vi "Load Plugins.vi"(8 "error in (no error)":errorcluster, 11 "Data in":T1) -> (0 "error out":errorcluster, 3 "Data out":T1)   [LabVIEW 2020]
uses:
  Type Definitions/Data.ctl
  Plugin Servers/Controller Array/Controller Array.lvclass
  Plugin Servers/Parameter to Hardware Map/Parameter to Hardware Map.lvclass
  <userlib>/RxnRover/DynamicReentrant/src/Type Defs/Message.ctl
  Plugin Manager/Plugin Details.ctl
  Plugin Servers/Controller/Controller Type.ctl
  Plugin Manager/Plugin Types.ctl
  Experiment/Experiment File/Experiment File Cluster.ctl
  Plugin Servers/Controller/Minimal Controller Cluster.ctl
  Plugin Servers/Parameter to Hardware Map/Minimal Map.ctl
  Plugin Servers/Parameter to Hardware Map/Minimal Pair Cluster.ctl
  Plugin Manager/Plugin Manager.lvlib
  <userlib>/RxnRover/DynamicReentrant/Dynamic Reentrant.lvlib
  Plugin Servers/Controller/Generic Plugin.lvclass
  Experiment/Experiment File/Experiment File.lvlib
panel:
  # "Note: Other controls and indicators are hidden!"
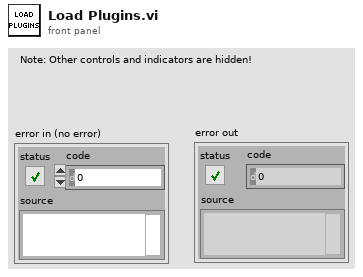
[diagram p1: front panel]
types:
  T1 = typedef "Data.ctl" = cluster{"Main VI Queue":refnum<queue>, "Process Queue References":refnum<queue>[], "Message Queue":refnum<queue>, "Visible Hardware VI":string, "Current Message":T2, "Message History":string[][], "Hardware":cluster{"Process Cache":refnum<class "Controller Array.lvclass">, "Plugins":T3[]}, "Optimizers":cluster{"Process Cache":refnum<class "Controller Array.lvclass">, "Plugins":T3[], "First parameters?":bool, "New Parameters":cluster{"Time Stamp":timestamp, "Names":string[], "Values":dbl[]}}, "Parameter to Hardware Map":refnum<class "Parameter to Hardware Map.lvclass">, "Analyzers":cluster{"Process Cache":refnum<class "Controller Array.lvclass">, "Plugins":T3[]}, "Log Directory":path, "Auto Pass Parameters":bool, "Experiment":cluster{"Name":string, "File Path":path, "File Extension":string, "File Cluster":T6}}
  T2 = typedef "Dynamic Reentrant.lvlib/Message.ctl" = cluster{"Source":string, "Destination":string, "Time Stamp":timestamp, "Command":string, "Data":variant}
  T3 = typedef "Plugin Manager.lvlib/Plugin Details.ctl" = cluster{"Plugin Name":string, "Controller Type":T4, "Control Panel Path":path, "Plugin Type":T5}
  T4 = typedef "Generic Plugin.lvclass/Controller Type.ctl" = enum16{"Invalid", "Temperature Controller", "Pump Controller", "Generic Optimizer", "LC Parser"}
  T5 = typedef "Plugin Manager.lvlib/Plugin Types.ctl" = enum16{"Invalid", "Optimizer", "Analyzer", "Hardware"}
  T6 = typedef "Experiment File.lvlib/Experiment File Cluster.ctl" = cluster{"Hardware List":T7[], "Optimizer List":T7[], "Analyzer List":T7[], "Parameter to Hardware Map":T8}
  T7 = typedef "Generic Plugin.lvclass/Minimal Controller Cluster.ctl" = cluster{"Name":string, "Controller Type":string, "Control Panel Path":string, "Resource":string}
  T8 = typedef "Parameter to Hardware Map.lvclass/Minimal Map.ctl" = T9[]
  T9 = typedef "Parameter to Hardware Map.lvclass/Minimal Pair Cluster.ctl" = cluster{"key":string, "values":T7[]}
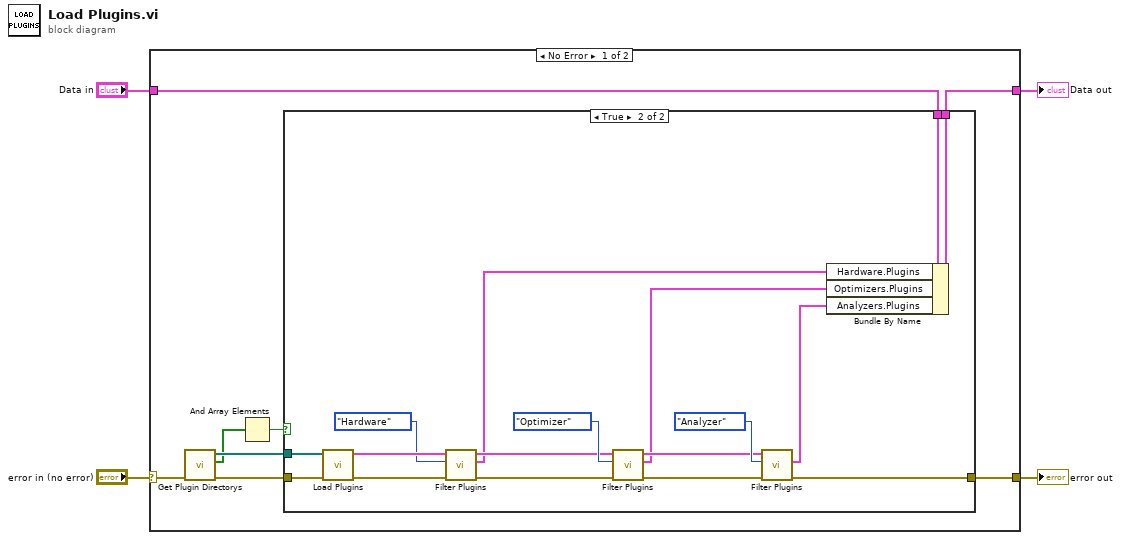
[diagram p0: block diagram]
diagram:
  n1 = case shown="No Error" "error in (no error)" {
    selector: "error in (no error)" -> [w12 w33]
    tunnel: [w6 w32] -> w4
    tunnel: "Data in" -> [w5 w32]
    tunnel: [w11 w33] -> w2
    frame No Error {
      n2 = call "Get Plugin Directorys.vi"("error in"=w12) -> ("error out"=w10:errorcluster, "Creation Success"=w7:bool[], "Plugin Directories"=w9:path[])  [unwired: 8 in]
      n3 = And Array Elements(Boolean array=w7) -> (logical AND=w8:bool)
      n4 = case shown="True" w8 {
        tunnel: [w14 w22] -> w11
        tunnel: w10 -> [w14 w31]
        tunnel: w9 -> [_ w30]
        tunnel: w5 -> [w13 w29]
        tunnel: [w13 w28] -> w6
        frame False {
        }
        frame True {
          n5 = call "Load Plugins.vi"("error in (no error)"=w31, "Plugin Directories"=w30) -> ("error out"=w26:errorcluster, "Plugin Array"=w27:T3[])  [unwired: 8 in]
          n6 = call "Filter Plugins.vi"("error in (no error)"=w26, "Plugin Type"=Plugin_Types."Hardware", "Full Plugin Array"=w27) -> ("error out"=w24:errorcluster, "Filtered Plugin Array out"=w17:T3[], "Full Plugin Array out (dup)"=w19:T3[])  [unwired: 6 in]
          n7 = call "Filter Plugins.vi"("error in (no error)"=w24, "Plugin Type"=Plugin_Types."Optimizer", "Full Plugin Array"=w19) -> ("error out"=w23:errorcluster, "Filtered Plugin Array out"=w16:T3[], "Full Plugin Array out (dup)"=w18:T3[])  [unwired: 6 in]
          n8 = call "Filter Plugins.vi"("error in (no error)"=w23, "Plugin Type"=Plugin_Types."Analyzer", "Full Plugin Array"=w18) -> ("error out"=w22:errorcluster, "Filtered Plugin Array out"=w15:T3[])  [unwired: 6 in, 1 out]
          n9 = Bundle By Name(cluster=w29, "Hardware.Plugins"=w17, "Optimizers.Plugins"=w16, "Analyzers.Plugins"=w15) -> (w28:T1)
        }
      }
    }
    frame Error {
    }
  }
  "Data out" <- w4
  "error out" <- w2
